vi "net方法-启动模拟器.vi"(10 "端口号":u16, 11 "vi索引":u16) -> (2 "错误输出":errorcluster)   [LabVIEW 2017]
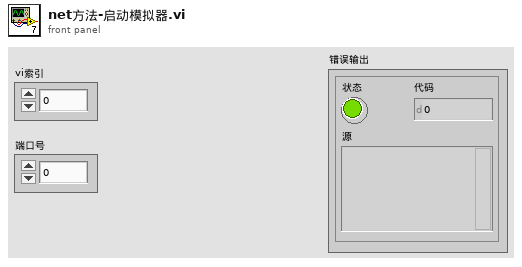
[diagram p1: front panel]
types:
  T1 = enum32{"Invalid", "Standard", "Closed", "Hidden", "Minimized", "Maximized"}
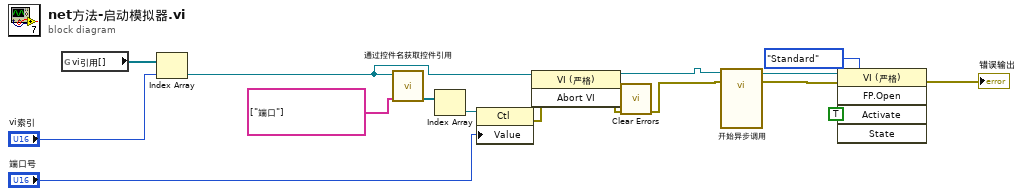
[diagram p0: block diagram]
diagram:
  n1 = global read "全局-模拟器变量.vi" "vi引用[]"() -> (w11:refnum<vi>[])
  n2 = Index Array(array=w11, index="vi索引") -> (element=w1:refnum<vi>)
  n3 = call "通过控件名获取控件引用.vi"("控件名数组"=string[] ["端口"], "VI引用"=w1) -> ("控件引用输出"=w15:refnum<vi>[])  [unwired: 7 in, 2 out]
  n4 = Index Array(array=w15) -> (element=w14:refnum<vi>)  [unwired: 1 in]
  n5 = property class="Ctl"(reference=w14, "Value"="端口号") -> (error out=w12:errorcluster)  [unwired: 1 in, 1 out]
  n6 = invoke class="VI (严格)" method="Abort VI"(reference=w1, error in=w12) -> (reference out=w5:refnum<vi>, error out=w9:errorcluster)  [unwired: 1 in, 1 out]
  n7 = call <vilib>:"Clear Errors.vi"("error in (no error)"=w9) -> ("error out"=w3:errorcluster)  [unwired: 5 in, 1 out]
  n8 = call-by-ref "开始异步调用"(reference=w5, error in=w3) -> (reference out=w4:refnum<vi>, error out=w2:errorcluster)  [unwired: 12 in]
  n9 = invoke class="VI (严格)" method="FP.Open"(reference=w4, error in=w2, "Activate"=TRUE ("激活？"), "State"=T1."Standard" ("状态")) -> (error out=→"错误输出":errorcluster)  [unwired: 1 in, 4 out]
